vi "Insert Start Message.vi"(8 "error in (no error)":errorcluster, 10 "Start Time":timestamp, 11 "Electrophysiology in":refnum<class "Electrophysiology.lvclass">) -> (0 "error out":errorcluster, 3 "Electrophysiology out":refnum<class "Electrophysiology.lvclass">)   [LabVIEW 2011, in "Electrophysiology.lvclass"]
uses:
  Electrophysiology.lvclass
  Database/EphysPrimary.ctl
  AcquireTraces/AcquireTraces.lvclass
  Database/SessionPrimary.ctl
  <vilib>/addons/database/NI_Database_API.lvlib
  AcquistionObject/AcquistionObject.lvclass
panel:
  out "EphysPK":T1
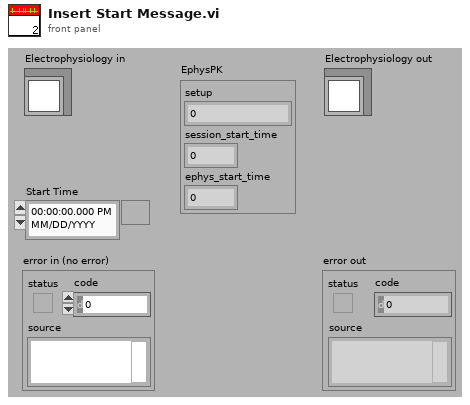
[diagram p1: front panel]
types:
  T1 = typedef "EphysPrimary.ctl" = cluster{"setup":u8, "session_start_time":dbl, "ephys_start_time":dbl}
  T2 = cluster{"setup":u8, "session_start_time":dbl, "ephys_start_time":dbl, "ephys_path":path}
  T3 = typedef "NI_Database_API.lvlib/Conn ObjectReference.ctl" = refnum<k1>
  T4 = typedef "SessionPrimary.ctl" = cluster{"setup":u8, "session_start_time":dbl}
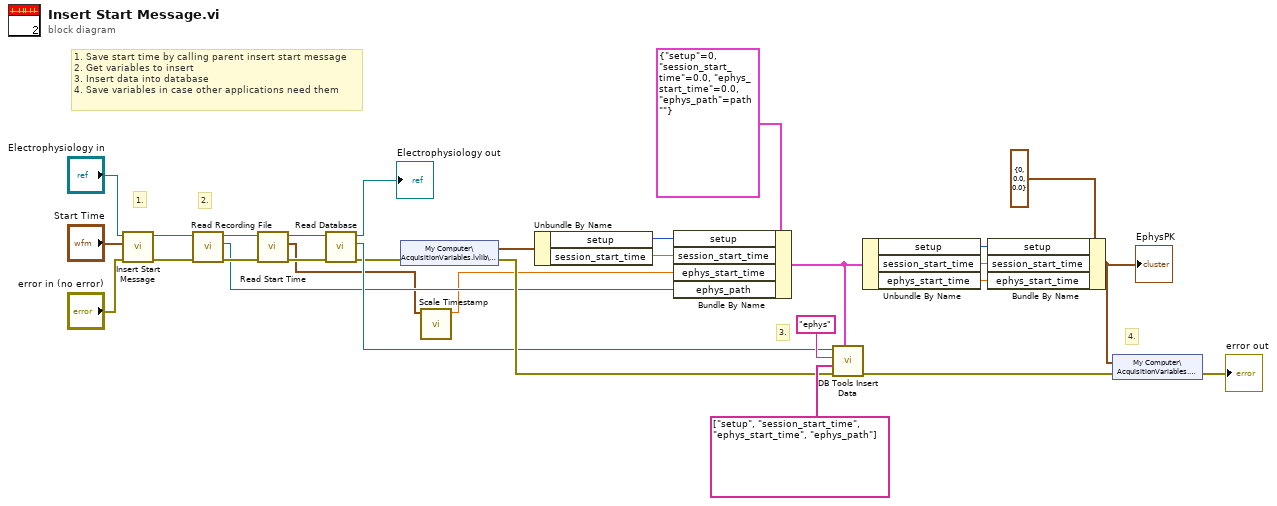
[diagram p0: block diagram]
diagram:
  # "4."
  # "2."
  # "3."
  # "1. Save start time by calling parent insert start message\n2. Get variables to insert\n3. Insert data into database\n4. Save variables in case other applications need them"
  # "1."
  n1 = call-parent "Insert Start Message.vi"("error in (no error)"="error in (no error)", "Start Time"="Start Time", "AcquireTraces in"="Electrophysiology in") -> ("error out"=w3:errorcluster, "AcquireTraces out"=w4:refnum<class "Electrophysiology.lvclass">)  [unwired: 7 in]
  n2 = call-dynamic "Read Recording File.vi"("error in (no error)"=w3, "AcquistionObject in"=w4) -> ("error out"=w12:errorcluster, "Recording File"=w7:path, "AcquistionObject out"=w13:refnum<class "Electrophysiology.lvclass">)  [unwired: 7 in]
  n3 = call-dynamic "Read Start Time.vi"("error in (no error)"=w12, "AcquistionObject in"=w13) -> ("error out"=w10:errorcluster, "Start Time"=w2:timestamp, "AcquistionObject out"=w11:refnum<class "Electrophysiology.lvclass">)  [unwired: 7 in]
  n4 = call-dynamic "Read Database.vi"("error in (no error)"=w10, "AcquistionObject in"=w11) -> ("error out"=w8:errorcluster, "reference"=w9:T3, "AcquistionObject out"=→"Electrophysiology out":refnum<class "Electrophysiology.lvclass">)  [unwired: 7 in]
  n5 = shared-variable "My Computer\\AcquisitionVariables.lvlib\\SessionPK"(error in=w8) -> (w17:T4, error out=w16:errorcluster)
  n6 = call "Scale Timestamp.vi"("Time Stamp"=w2) -> ("Scaled timestamp"=w1:dbl)  [unwired: 10 in]
  n7 = Unbundle By Name(w17) -> ("setup"=w24:u8, "session_start_time"=w23:dbl)
  n8 = Bundle By Name(cluster=T2 {"setup"=0, "session_start_time"=0.0, "ephys_start_time"=0.0, "ephys_path"=path ""} ("Cluster"), "setup"=w24, "session_start_time"=w23, "ephys_start_time"=w1, "ephys_path"=w7) -> (w21:T2)
  n9 = call <vilib>:"DB Tools Insert Data.vi"("data"=w21, "error in (no error)"=w16, "columns"=string[] ["setup", "session_start_time", "ephys_start_time", "ephys_path"], "table"="ephys", "connection reference"=w9) -> ("error out"=w14:errorcluster)  [unwired: 5 in, 1 out]
  n10 = Unbundle By Name(w21) -> ("setup"=w20:u8, "session_start_time"=w19:dbl, "ephys_start_time"=w18:dbl)
  n11 = Bundle By Name(cluster=T1 {"setup"=0, "session_start_time"=0.0, "ephys_start_time"=0.0} ("EphysPK"), "setup"=w20, "session_start_time"=w19, "ephys_start_time"=w18) -> (w15:T1)
  "EphysPK" <- w15
  n12 = shared-variable "My Computer\\AcquisitionVariables.lvlib\\EphysPK"(w15, error in=w14) -> (error out=→"error out":errorcluster)
